vi "CALC_Coordinates_Diff_R_Center_(offline).vi"(3 "Error In":errorcluster, 4 "Frame time, s":dbl=0.0125, 5 "Magnets coordinates in":dbl[][](array[numeric])) -> (0 "Error Out":errorcluster, 2 "Output cluster of data":T1)   [LabVIEW 2018, in "Tracker.lvlib"]
uses:
  Tracker.lvlib
  Controls/CTL_Cage_Coords_(arrays).ctl
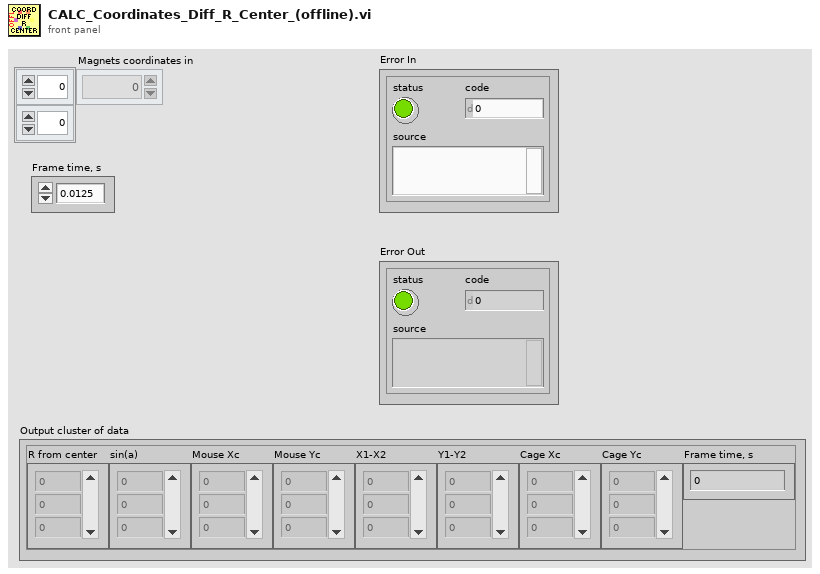
[diagram p1: front panel]
types:
  T1 = typedef "Tracker.lvlib/CTL_Cage_Coords_(arrays).ctl" = cluster{"R from center":dbl[], "sin(a)":dbl[], "Mouse Xc":dbl[], "Mouse Yc":dbl[], "X1-X2":dbl[], "Y1-Y2":dbl[], "Cage Xc":dbl[], "Cage Yc":dbl[], "Frame time, s":dbl}
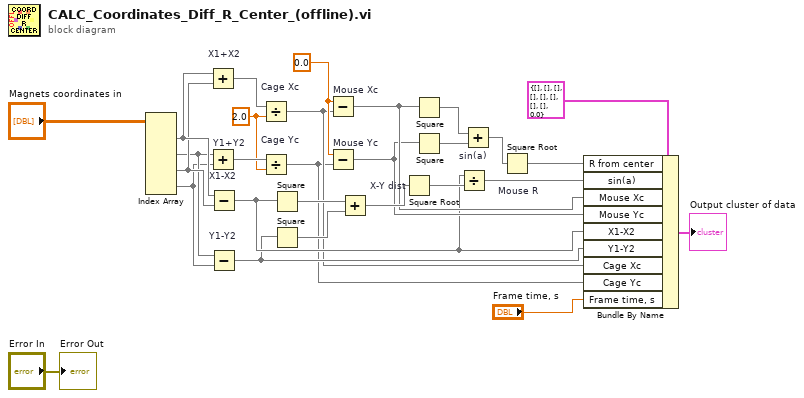
[diagram p0: block diagram]
diagram:
  w19 = 0.0
  w20 = 2.0
  n1 = Index Array(array="Magnets coordinates in") -> (element #1=w26:dbl[], element #2=w24:dbl[], element #3=w25:dbl[], element #4=w23:dbl[])  [unwired: 8 in]
  n2 = Add "X1+X2"(x=w26, y=w25) -> (x+y=w22:dbl[])
  n3 = Add "Y1+Y2"(x=w24, y=w23) -> (x+y=w21:dbl[])
  n4 = Subtract "X1-X2"(x=w26, y=w25) -> (x-y=w6:dbl[])
  n5 = Subtract "Y1-Y2"(x=w24, y=w23) -> (x-y=w5:dbl[])
  n6 = Divide "Cage Xc"(x=w22, y=w20) -> (x/y=w4:dbl[])
  n7 = Divide "Cage Yc"(x=w21, y=w20) -> (x/y=w3:dbl[])
  n8 = Square(x=w6) -> (x^2=w17:dbl[])
  n9 = Square(x=w5) -> (x^2=w16:dbl[])
  n10 = Subtract "Mouse Xc"(x=w19, y=w4) -> (x-y=w8:dbl[])
  n11 = Subtract "Mouse Yc"(x=w19, y=w3) -> (x-y=w7:dbl[])
  n12 = Add(x=w17, y=w16) -> (x+y=w18:dbl[])
  n13 = Square Root "X-Y dist"(x=w18) -> (sqrt(x)=w12:dbl[])
  n14 = Square(x=w8) -> (x^2=w15:dbl[])
  n15 = Square(x=w7) -> (x^2=w14:dbl[])
  n16 = Divide "sin(a)"(x=w6, y=w12) -> (x/y=w9:dbl[])
  n17 = Add(x=w15, y=w14) -> (x+y=w13:dbl[])
  n18 = Square Root "Mouse R"(x=w13) -> (sqrt(x)=w10:dbl[])
  n19 = Bundle By Name(cluster=T1 {"R from center"=[], "sin(a)"=[], "Mouse Xc"=[], "Mouse Yc"=[], "X1-X2"=[], "Y1-Y2"=[], "Cage Xc"=[], "Cage Yc"=[], "Frame time, s"=0.0} ("Cage coords data"), "R from center"=w10, "sin(a)"=w9, "Mouse Xc"=w8, "Mouse Yc"=w7, "X1-X2"=w6, "Y1-Y2"=w5, "Cage Xc"=w4, "Cage Yc"=w3, "Frame time, s"="Frame time, s") -> (→"Output cluster of data":T1)
  "Error Out" <- "Error In"
